vi "reportTaskInit.vi"(7 "TaskRef":refnum<vi>, 8 "error in (no error)":errorcluster, 11 "pdbm_taskroute_feedback_event":refnum<user-event>) -> (0 "error out":errorcluster, 3 "pdbm_taskroute_feedback_event out":refnum<user-event>, 5 "TaskRef out":refnum<vi>)   [LabVIEW 2015, in "pdbm_tasks.lvlib"]
uses:
  pdbm_tasks.lvlib
  pdbm_test_route/UsrDefine/TaskFeedbackCmd.ctl
  pdbm_test_route/pdbm_task_route.lvlib
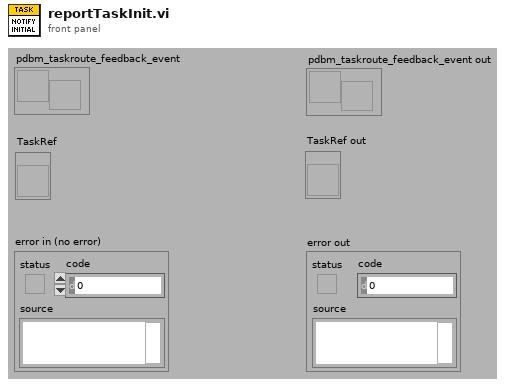
[diagram p1: front panel]
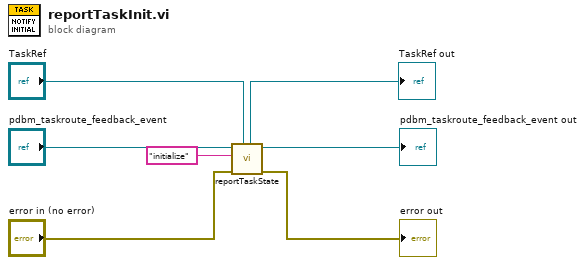
[diagram p0: block diagram]
diagram:
  n1 = call "reportTaskState.vi"("TaskRef"="TaskRef", "error in (no error)"="error in (no error)", "Request"="initialize", "pdbm_taskroute_feedback_event"="pdbm_taskroute_feedback_event") -> ("error out"=→"error out":errorcluster, "pdbm_taskroute_feedback_event out"=→"pdbm_taskroute_feedback_event out":refnum<user-event>, "TaskRef out"=→"TaskRef out":refnum<vi>)  [unwired: 5 in]
